vi "Build Report.vi"(8 "error in (no error)":errorcluster, 9 "Results":T1[](array[typedef]), 10 "Path":path, 11 "Macro in":refnum<class "Macro.lvclass">) -> (0 "error out":errorcluster, 3 "Macro out":refnum<class "Macro.lvclass">)   [LabVIEW 2020, in "MacroAssert.lvlib" / "Macro.lvclass"]
doc: "Builds a report consisting of the actions and assertions performed and associated <B>Results</B> and saves it to <B>Path</B>."
uses:
  Macro.lvclass
  CTLs/Result.ctl
  CTLs/Outcome.ctl
  <vilib>/Utility/NIReport.llb/Report Type.ctl
  Macro.lvclass/Macro.ctl
  <vilib>/Utility/NIReport.llb/Append Report Text (str wrap).vi
  <vilib>/Utility/NIReport.llb/NI_report.lvclass
  Step/Step.lvclass
  <vilib>/Utility/NIReport.llb/NI_ReportGenerationCore.lvlib
  MacroAssert.lvlib
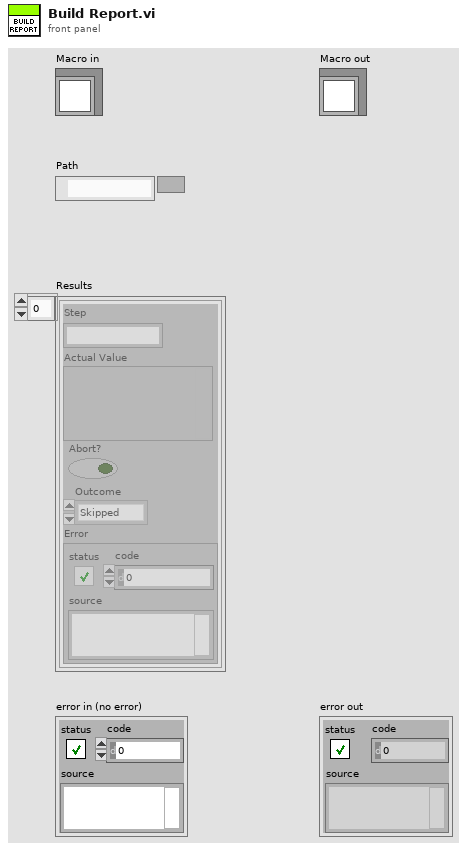
[diagram p1: front panel]
types:
  T1 = typedef "MacroAssert.lvlib/Result.ctl" = cluster{"Step":string, "Actual Value":variant, "Abort?":bool, "Outcome":T2, "Error":errorcluster}
  T2 = typedef "MacroAssert.lvlib/Outcome.ctl" = enum16{"Not Started", "Skipped", "Pass", "Fail", "Complete", "Error", "Auto Abort", "User Abort"}
  T3 = typedef "NI_ReportGenerationCore.lvlib/Report Type.ctl" = enum16{"HTML", "Word", "Excel"}
  T4 = typedef "MacroAssert.lvlib/Macro Config v1.ctl" = cluster{"Schema Version":string, "N":i32, "Description":string, "Resolutions":cluster{"Width":i16, "Height":i16}[], "Date Created":timestamp, "Date Updated":timestamp}
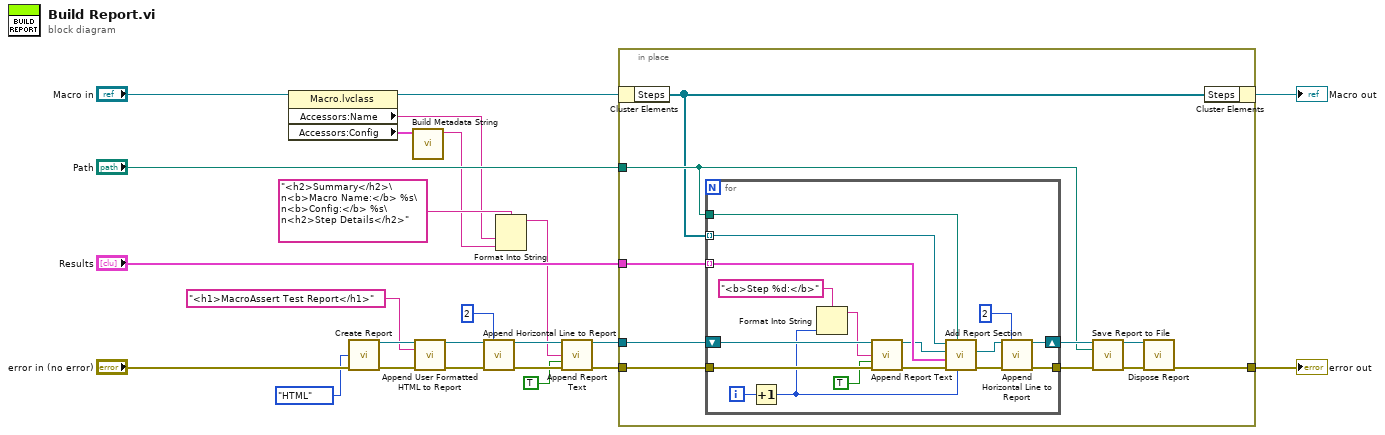
[diagram p0: block diagram]
diagram:
  n1 = property class="Macro.lvclass"(reference="Macro in") -> (reference out=w13:refnum<class "Macro.lvclass">, "Accessors:Name"=w4:string, "Accessors:Config"=w6:T4)  [unwired: 1 in, 1 out]
  n2 = call <vilib>:"Create Report.vi"("report type"=Report_Type."HTML", "error in (no error)"="error in (no error)") -> ("report out"=w14:refnum<class "NI_report.lvclass">, "error out"=w22:errorcluster)  [unwired: 12 in]
  n3 = call "Build Metadata String.vi"("Macro Config"=w6) -> ("Metadata"=w5:string)  [unwired: 10 in]
  n4 = call-dynamic "Append User Formatted HTML to Report.vi"("report in"=w14, "HTML text"="<h1>MacroAssert Test Report</h1>", "error in (no error)"=w22) -> ("report out"=w10:refnum<class "NI_report.lvclass">, "error out"=w21:errorcluster)  [unwired: 11 in]
  n5 = call-dynamic "Append Horizontal Line to Report.vi"("report in"=w10, "size (default)"=2, "error in (no error)"=w21) -> ("report out"=w8:refnum<class "NI_report.lvclass">, "error out"=w20:errorcluster)  [unwired: 11 in]
  n6 = Format Into String(format string="<h2>Summary</h2>\n<b>Macro Name:</b> %s\n<b>Config:</b> %s\n<h2>Step Details</h2>", w4, w5) -> (resulting string=w3:string)  [unwired: 2 in, 1 out]
  n7 = call-poly <vilib>:"Append Report Text.vi"("report in"=w8, "text"=w3, "append on new line? (F)"=TRUE, "error in (no error)"=w20) -> ("report out"=w1:refnum<class "NI_report.lvclass">, "error out"=w2:errorcluster)  [unwired: 8 in, 2 out]
  n8 = in-place {
    in-place-border: "Path" -> [w28]
    in-place-border: [w33] -> w24
    in-place-border: "Results" -> [w26]
    in-place-border: w2 -> [w31]
    in-place-border: w1 -> [w25]
    n9 = in-place-cluster #1(w13) -> ("Steps"=w27:refnum<class "Step.lvclass">[])
    n10 = for {
      tunnel: w31 -> [w49]
      tunnel: w27 -> [w46] mode=indexing
      tunnel: w26 -> [w45] mode=indexing
      tunnel: [w50] -> w32
      shift-right: [w44] -> w29
      shift-left: w25 -> [w40]
      tunnel: w28 -> [w42]
      i -> [w43]
      n11 = Increment(x=w43) -> (x+1=w37:i32)
      n12 = Format Into String(format string="<b>Step %d:</b>", w37) -> (resulting string=w36:string)  [unwired: 2 in, 1 out]
      n13 = call-poly <vilib>:"Append Report Text.vi"("report in"=w40, "text"=w36, "append on new line? (F)"=TRUE, "error in (no error)"=w49) -> ("report out"=w35:refnum<class "NI_report.lvclass">, "error out"=w48:errorcluster)  [unwired: 8 in, 2 out]
      n14 = call-dynamic "Add Report Section.vi"("Step Number"=w37, "Report Path"=w42, "error in (no error)"=w48, "Result"=w45, "Report in"=w35, "Step in"=w46) -> ("error out"=w51:errorcluster, "Report out"=w47:refnum<class "NI_report.lvclass">)  [unwired: 3 in, 1 out]
      n15 = call-dynamic "Append Horizontal Line to Report.vi"("report in"=w47, "size (default)"=2, "error in (no error)"=w51) -> ("report out"=w44:refnum<class "NI_report.lvclass">, "error out"=w50:errorcluster)  [unwired: 11 in]
    }
    n16 = call-dynamic "Save Report to File.vi"("report in"=w29, "report file path"=w28, "error in (no error)"=w32) -> ("report out"=w30:refnum<class "NI_report.lvclass">, "error out"=w34:errorcluster)  [unwired: 11 in]
    n17 = call-dynamic "Dispose Report.vi"("report in"=w30, "error in (no error)"=w34) -> ("error out"=w33:errorcluster)  [unwired: 13 in]
    n18 = in-place-cluster #1("Steps"=w27) -> (→"Macro out":refnum<class "Macro.lvclass">)
  }
  "error out" <- w24
